vi "Set Parameters.vi"(8 "error in (no error)":errorcluster, 11 "Cluster in":T1={"Queue Array"=[], "Queue Element"={"state"="", "data"=variant}, "System Event"=refnum, "System Event RefNum"=refnum, "Queue List"=[], "LPCA COM"="", "Rotating"=FALSE, "PrecorAI"="", "T_0 Index"=0, "Bar Graph X"=[], "Channels"=[], "Active Indicies"=[], "Active Channels"=[], "Sample Frequency"=0.0, "Ibrake Sweep"=[], "RPM Sweep"=[], "Load Sweep"=[], "Step Height Sweep"=[], "Range Sweep"=[], "A Counter"=0, "B Counter"=0, "C Counter"=0, "#A"=0, "#B"=0, "#C"=0, "Current RPM"=0.0, "Current Ibrake"=0, "Current Range"=0, "Current Step Height"=0, "Load Bank"=enum."OFF", "Cfg Cntrls"=[], "T_Monitor Indices"=[], "Thermal Limit"=0, "Thermal Resume"=0, "Timer Reset"=FALSE, "Stop Time"=0.0, "Autotest"=FALSE, "Pulsed RPM Capture"=FALSE, "Get Sample"=FALSE, "Last State"="", "Reset Timeout"=FALSE, "Ctrl Refs"={"Test Details"=refnum, "Save Config"=refnum, "Load Config"=refnum, "Path"=refnum, "Snapshot"=refnum, "SS#"=refnum, "Ibrake"=refnum, "RPM Target"=refnum, "Spin"=refnum, "Load Bank"=refnum, "Start Test"=refnum, "Pause Test"=refnum, "Load Sweep"=refnum, "RPM Sweep"=refnum, "Ibrake Sweep"=refnum, "Filters"=refnum, "Sample Frequency"=refnum, "Data Setup"=refnum, "Pause"=refnum, "Stop Time"=refnum, "S Period"=refnum, "Range"=refnum, "Step Height"=refnum, "Step Height Sweep"=refnum, "Range Sweep"=refnum, "Available Tests"=refnum, "RPM Graph"=refnum, "RPM Knob"=refnum, "FanMode"=refnum, "Fan Mode LED Array"=refnum, "Thermal Equilibrium"=refnum, "Data Display"=refnum, "LPCA Error"=refnum, "LPCA Ramp"=refnum, "LPCA Range"=refnum, "LPCA Resistance"=refnum, "Analyze Read"=refnum, "Console Select"=refnum, "Sub Panel"=refnum}, "Pulse Waveform"={"t0"=timestamp(0 s since 1904-01-01), "dt"=1.0, "Y"=[]}, "Snapshot"={"Test Details"="test", "Version"="test", "Date"=timestamp(3493915594.3018084 s since 1904-01-01), "Selected Test"="man", "Snapshot Number"=0, "Time"=timestamp(3493915602.7292905 s since 1904-01-01), "Ibrake Setpoint"="1", "RPM Setpoint"="20", "Range Setpoint"="", "Step Height Setpoint"="", "Load Bank Setpoint"="15", "Measurement Headers"="a,b,c,1,2,3", "Measurements"="1,2,3,4,5,6,7,8", "A"=0, "B"=0, "C"=0, "Raw Data"=[], "Available Tests"=enum."Manual", "Ibrake List"="", "RPM List"="", "Load Bank List"="", "Range List"="", "Step Height List"="", "FanMode Setpoint"=enum."Auto"}, "Sample Period"=0.0, "OverTemp"=FALSE, "Available Tests"=enum."Manual", "FanMode"=enum."Auto", "Fan Mode LED Array"=[FALSE, TRUE, FALSE], "Thermal\nEquilibrium "=FALSE, "Equilibrium Stop"=FALSE, "AvgDegChg"=[]} {"Snapshot"."Time" format="%<%H:%M:%S>T"; "Snapshot"."Date" format="%<%m/%d/%Y>T"}) -> (0 "error out":errorcluster, 3 "Cluster out":T1={"Queue Array"=[], "Queue Element"={"state"="", "data"=variant}, "System Event"=refnum, "System Event RefNum"=refnum, "Queue List"=[], "LPCA COM"="", "Rotating"=FALSE, "PrecorAI"="", "T_0 Index"=0, "Bar Graph X"=[], "Channels"=[], "Active Indicies"=[], "Active Channels"=[], "Sample Frequency"=0.0, "Ibrake Sweep"=[], "RPM Sweep"=[], "Load Sweep"=[], "Step Height Sweep"=[], "Range Sweep"=[], "A Counter"=0, "B Counter"=0, "C Counter"=0, "#A"=0, "#B"=0, "#C"=0, "Current RPM"=0.0, "Current Ibrake"=0, "Current Range"=0, "Current Step Height"=0, "Load Bank"=enum."OFF", "Cfg Cntrls"=[], "T_Monitor Indices"=[], "Thermal Limit"=0, "Thermal Resume"=0, "Timer Reset"=FALSE, "Stop Time"=0.0, "Autotest"=FALSE, "Pulsed RPM Capture"=FALSE, "Get Sample"=FALSE, "Last State"="", "Reset Timeout"=FALSE, "Ctrl Refs"={"Test Details"=refnum, "Save Config"=refnum, "Load Config"=refnum, "Path"=refnum, "Snapshot"=refnum, "SS#"=refnum, "Ibrake"=refnum, "RPM Target"=refnum, "Spin"=refnum, "Load Bank"=refnum, "Start Test"=refnum, "Pause Test"=refnum, "Load Sweep"=refnum, "RPM Sweep"=refnum, "Ibrake Sweep"=refnum, "Filters"=refnum, "Sample Frequency"=refnum, "Data Setup"=refnum, "Pause"=refnum, "Stop Time"=refnum, "S Period"=refnum, "Range"=refnum, "Step Height"=refnum, "Step Height Sweep"=refnum, "Range Sweep"=refnum, "Available Tests"=refnum, "RPM Graph"=refnum, "RPM Knob"=refnum, "FanMode"=refnum, "Fan Mode LED Array"=refnum, "Thermal Equilibrium"=refnum, "Data Display"=refnum, "LPCA Error"=refnum, "LPCA Ramp"=refnum, "LPCA Range"=refnum, "LPCA Resistance"=refnum, "Analyze Read"=refnum, "Console Select"=refnum, "Sub Panel"=refnum}, "Pulse Waveform"={"t0"=timestamp(0 s since 1904-01-01), "dt"=1.0, "Y"=[]}, "Snapshot"={"Test Details"="test", "Version"="test", "Date"=timestamp(3493915594.3018084 s since 1904-01-01), "Selected Test"="man", "Snapshot Number"=0, "Time"=timestamp(3493915602.7292905 s since 1904-01-01), "Ibrake Setpoint"="1", "RPM Setpoint"="20", "Range Setpoint"="", "Step Height Setpoint"="", "Load Bank Setpoint"="15", "Measurement Headers"="a,b,c,1,2,3", "Measurements"="1,2,3,4,5,6,7,8", "A"=0, "B"=0, "C"=0, "Raw Data"=[], "Available Tests"=enum."Manual", "Ibrake List"="", "RPM List"="", "Load Bank List"="", "Range List"="", "Step Height List"="", "FanMode Setpoint"=enum."Auto"}, "Sample Period"=0.0, "OverTemp"=FALSE, "Available Tests"=enum."Manual", "FanMode"=enum."Auto", "Fan Mode LED Array"=[FALSE, TRUE, FALSE], "Thermal\nEquilibrium "=FALSE, "Equilibrium Stop"=FALSE, "AvgDegChg"=[]} {"Snapshot"."Time" format="%<%H:%M:%S>T"; "Snapshot"."Date" format="%<%m/%d/%Y>T"})   [LabVIEW 2017]
uses:
  Controls/Test TypeDef.ctl
  Code Library/Queue References Array.ctl
  Code Library/Queue Element.ctl
  Controls/Load Bank.ctl
  Controls/Available Tests.ctl
  Console Sim/Controls/Console Select.ctl
  Controls/Snapshot Typedef.ctl
  Controls/FanMode.ctl
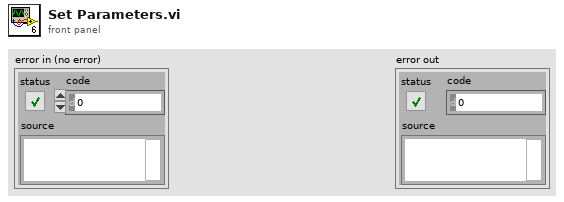
[diagram p1: front panel]
types:
  T1 = typedef "Test TypeDef.ctl" = cluster{"Queue Array":T2, "Queue Element":T3, "System Event":refnum<user-event>, "System Event RefNum":refnum<event-registration>, "Queue List":string[], "LPCA COM":refnum<visa-resource-name>, "Rotating":bool, "PrecorAI":refnum<k21>, "T_0 Index":i32, "Bar Graph X":i32[], "Channels":string[], "Active Indicies":i32[], "Active Channels":string[][], "Sample Frequency":dbl, "Ibrake Sweep":string[], "RPM Sweep":string[], "Load Sweep":string[], "Step Height Sweep":string[], "Range Sweep":string[], "A Counter":i32, "B Counter":i32, "C Counter":i32, "#A":i32, "#B":i32, "#C":i32, "Current RPM":dbl, "Current Ibrake":u32, "Current Range":u32, "Current Step Height":u32, "Load Bank":T4, "Cfg Cntrls":refnum<vi>[], "T_Monitor Indices":i32[], "Thermal Limit":i32, "Thermal Resume":i32, "Timer Reset":bool, "Stop Time":dbl, "Autotest":bool, "Pulsed RPM Capture":bool, "Get Sample":bool, "Last State":string, "Reset Timeout":bool, "Ctrl Refs":cluster{"Test Details":refnum<vi>, "Save Config":refnum<vi>, "Load Config":refnum<vi>, "Path":refnum<vi>, "Snapshot":refnum<vi>, "SS#":refnum<vi>, "Ibrake":refnum<vi>, "RPM Target":refnum<vi>, "Spin":refnum<vi>, "Load Bank":refnum<vi>, "Start Test":refnum<vi>, "Pause Test":refnum<vi>, "Load Sweep":refnum<vi>, "RPM Sweep":refnum<vi>, "Ibrake Sweep":refnum<vi>, "Filters":refnum<vi>, "Sample Frequency":refnum<vi>, "Data Setup":refnum<vi>, "Pause":refnum<vi>, "Stop Time":refnum<vi>, "S Period":refnum<vi>, "Range":refnum<vi>, "Step Height":refnum<vi>, "Step Height Sweep":refnum<vi>, "Range Sweep":refnum<vi>, "Available Tests":refnum<vi>, "RPM Graph":refnum<vi>, "RPM Knob":refnum<vi>, "FanMode":refnum<vi>, "Fan Mode LED Array":refnum<vi>, "Thermal Equilibrium":refnum<vi>, "Data Display":refnum<vi>, "LPCA Error":refnum<vi>, "LPCA Ramp":refnum<vi>, "LPCA Range":refnum<vi>, "LPCA Resistance":refnum<vi>, "Analyze Read":refnum<vi>, "Console Select":refnum<vi>, "Sub Panel":refnum<vi>}, "Pulse Waveform":waveform(dbl), "Snapshot":T5, "Sample Period":dbl, "OverTemp":bool, "Available Tests":T6, "FanMode":T7, "Fan Mode LED Array":bool[], "Thermal\nEquilibrium ":bool, "Equilibrium Stop":bool, "AvgDegChg":dbl[]}
  T2 = typedef "Queue References Array.ctl" = refnum<queue>[]
  T3 = typedef "Queue Element.ctl" = cluster{"state":string, "data":variant}
  T4 = typedef "Load Bank.ctl" = enum16{"OFF", "50", "25", "16.7", "12.5", "10.0", "8.3", "7.1", "6.3", "5.6", "5.0", "4.5", "4.2", "3.8", "3.6", "3.3", "3.1"}
  T5 = typedef "Snapshot Typedef.ctl" = cluster{"Test Details":string, "Version":string, "Date":timestamp, "Selected Test":string, "Snapshot Number":u16, "Time":timestamp, "Ibrake Setpoint":string, "RPM Setpoint":string, "Range Setpoint":string, "Step Height Setpoint":string, "Load Bank Setpoint":string, "Measurement Headers":string, "Measurements":string, "A":i32, "B":i32, "C":i32, "Raw Data":string[][], "Available Tests":T6, "Ibrake List":string, "RPM List":string, "Load Bank List":string, "Range List":string, "Step Height List":string, "FanMode Setpoint":T7}
  T6 = typedef "Available Tests.ctl" = enum16{"Manual", "EFX Brake Torque", "Generator Torque", "EFX Brake Thermal", "Generator Thermal", "Pulsed RPM", "AMT Brake Torque", "Bike Brake Torque", "AMT Brake Thermal", "Bike Brake Thermal"}
  T7 = typedef "FanMode.ctl" = enum16{"On", "Off", "Auto"}
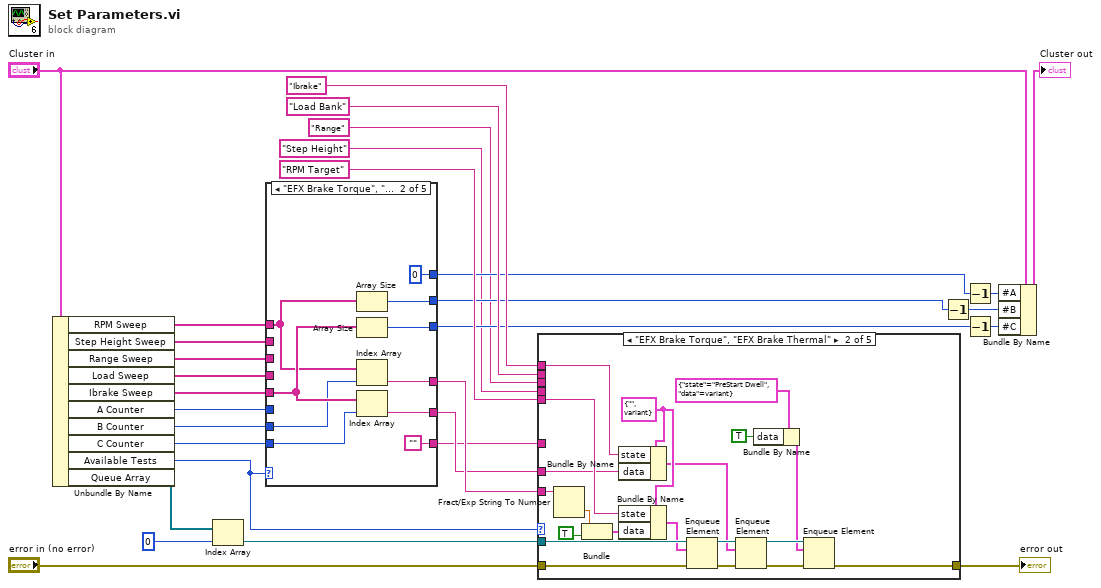
[diagram p0: block diagram]
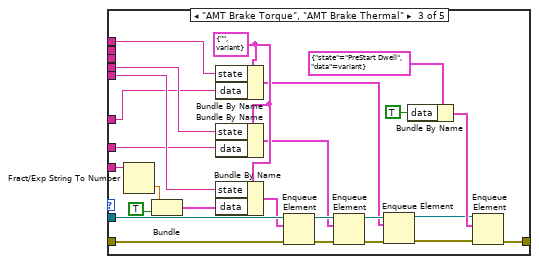
[diagram p3: hidden frame]
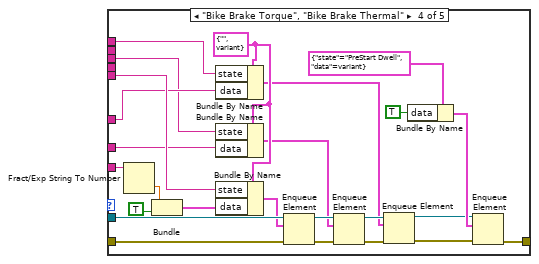
[diagram p4: hidden frame]
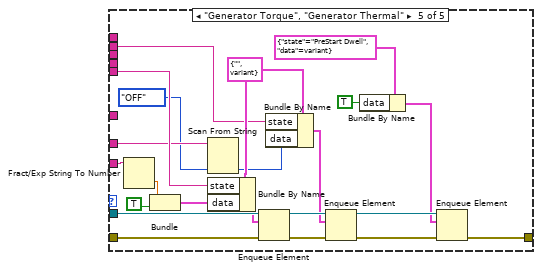
[diagram p5: hidden frame]
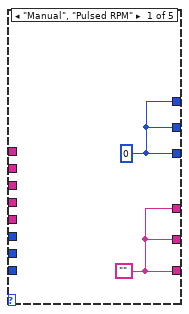
[diagram p6: hidden frame]
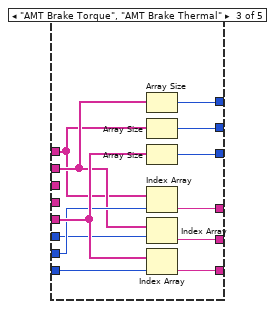
[diagram p7: hidden frame]
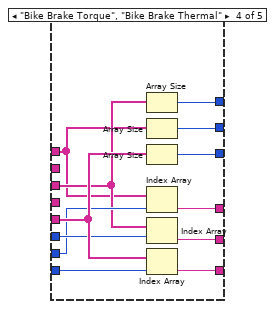
[diagram p8: hidden frame]
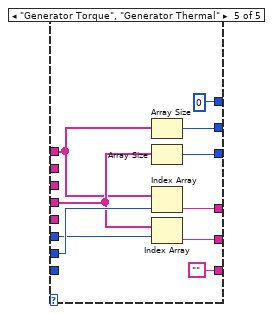
[diagram p9: hidden frame]
diagram:
  n1 = Unbundle By Name("Cluster in") -> ("RPM Sweep"=w19:string[], "Step Height Sweep"=w20:string[], "Range Sweep"=w21:string[], "Load Sweep"=w11:string[], "Ibrake Sweep"=w10:string[], "A Counter"=w17:i32, "B Counter"=w18:i32, "C Counter"=w9:i32, "Available Tests"=w26:T6, "Queue Array"=w24:T2)
  n2 = Index Array(array=w24, index=0) -> (element=w25:refnum<queue>)
  n3 = case shown="\"EFX Brake Torque\", \"EFX Brake Thermal\"" w26 {
    tunnel: w19 -> [_ w39 w46 w55 w71]
    tunnel: w20 -> [_ _ w47 _ _]
    tunnel: w21 -> [_ _ _ w56 _]
    tunnel: w17 -> [_ _ w48 w58 w73]
    tunnel: w18 -> [_ w34 w49 w57 w74]
    tunnel: [w32 w41 w54 w66 w75] -> w2
    tunnel: [w32 w42 w53 w65 w76] -> w3
    tunnel: [w31 w37 w45 w64 w69] -> w7
    tunnel: [w31 0 w43 w63 0] -> w6
    tunnel: w11 -> [_ _ _ _ w72]
    tunnel: w10 -> [_ w40 w51 w61 _]
    tunnel: w9 -> [_ w33 w52 w62 _]
    tunnel: [w31 w36 w44 w60 w68] -> w8
    tunnel: [w32 "" w50 w59 ""] -> w1
    frame "Manual", "Pulsed RPM" {
      w31 = 0
      w32 = ""
    }
    frame "EFX Brake Torque", "EFX Brake Thermal" {
      n4 = Array Size(array=w39) -> (size(s)=w37:i32)
      n5 = Array Size(array=w40) -> (size(s)=w36:i32)
      n6 = Index Array(array=w39, index=w34) -> (element=w42:string)
      n7 = Index Array(array=w40, index=w33) -> (element=w41:string)
    }
    frame "AMT Brake Torque", "AMT Brake Thermal" {
      n8 = Array Size(array=w47) -> (size(s)=w43:i32)
      n9 = Array Size(array=w46) -> (size(s)=w45:i32)
      n10 = Array Size(array=w51) -> (size(s)=w44:i32)
      n11 = Index Array(array=w46, index=w49) -> (element=w53:string)
      n12 = Index Array(array=w47, index=w48) -> (element=w54:string)
      n13 = Index Array(array=w51, index=w52) -> (element=w50:string)
    }
    frame "Bike Brake Torque", "Bike Brake Thermal" {
      n14 = Array Size(array=w56) -> (size(s)=w63:i32)
      n15 = Array Size(array=w55) -> (size(s)=w64:i32)
      n16 = Array Size(array=w61) -> (size(s)=w60:i32)
      n17 = Index Array(array=w55, index=w57) -> (element=w65:string)
      n18 = Index Array(array=w56, index=w58) -> (element=w66:string)
      n19 = Index Array(array=w61, index=w62) -> (element=w59:string)
    }
    frame "Generator Torque", "Generator Thermal" {
      n20 = Array Size(array=w71) -> (size(s)=w69:i32)
      n21 = Array Size(array=w72) -> (size(s)=w68:i32)
      n22 = Index Array(array=w71, index=w74) -> (element=w76:string)
      n23 = Index Array(array=w72, index=w73) -> (element=w75:string)
    }
  }
  n24 = case shown="\"EFX Brake Torque\", \"EFX Brake Thermal\"" w26 {
    tunnel: "error in (no error)" -> [w77 w96 w121 w146 w168]
    tunnel: [w77 w81 w111 w136 w153] -> w13
    tunnel: w25 -> [_ w95 w120 w145 w167]
    tunnel: "RPM Target" -> [_ w92 w117 w142 w164]
    tunnel: w3 -> [_ w91 w116 w141 w163]
    tunnel: "Load Bank" -> [_ _ _ _ w160]
    tunnel: w2 -> [_ w88 w104 w129 w156]
    tunnel: "Ibrake" -> [_ w84 w112 w137 _]
    tunnel: "Step Height" -> [_ _ w102 _ _]
    tunnel: "Range" -> [_ _ _ w123 _]
    tunnel: w1 -> [_ _ w101 w127 _]
    frame "Manual", "Pulsed RPM" {
    }
    frame "EFX Brake Torque", "EFX Brake Thermal" {
      w90 = T3 {"state"="", "data"=variant} ("element")
      n25 = Fract/Exp String To Number(string=w91) -> (number=w85:dbl)  [unwired: 3 in, 1 out]
      n26 = Bundle(w85, TRUE) -> (w87:cluster{dbl, bool})  [unwired: 1 in]
      n27 = Bundle By Name(cluster=w90, "state"=w84, "data"=w88) -> (w89:T3)
      n28 = Bundle By Name(cluster=w90, "state"=w92, "data"=w87) -> (w93:T3)
      n29 = Enqueue Element(queue=w95, element=w93, error in (no error)=w96) -> (queue out=w94:refnum<queue>, error out=w97:errorcluster)  [unwired: 1 in, 1 out]
      n30 = Enqueue Element(queue=w94, element=w89, error in (no error)=w97) -> (queue out=w83:refnum<queue>, error out=w82:errorcluster)  [unwired: 1 in, 1 out]
      n31 = Bundle By Name(cluster=T3 {"state"="PreStart Dwell", "data"=variant} ("element"), "data"=TRUE) -> (w79:T3)
      n32 = Enqueue Element(queue=w83, element=w79, error in (no error)=w82) -> (error out=w81:errorcluster)  [unwired: 1 in, 2 out]
    }
    frame "AMT Brake Torque", "AMT Brake Thermal" {
      w105 = T3 {"state"="", "data"=variant} ("element")
      n33 = Fract/Exp String To Number(string=w116) -> (number=w113:dbl)  [unwired: 3 in, 1 out]
      n34 = Bundle(w113, TRUE) -> (w115:cluster{dbl, bool})  [unwired: 1 in]
      n35 = Bundle By Name(cluster=w105, "state"=w112, "data"=w101) -> (w100:T3)
      n36 = Bundle By Name(cluster=w105, "state"=w102, "data"=w104) -> (w103:T3)
      n37 = Bundle By Name(cluster=w105, "state"=w117, "data"=w115) -> (w118:T3)
      n38 = Enqueue Element(queue=w120, element=w118, error in (no error)=w121) -> (queue out=w119:refnum<queue>, error out=w122:errorcluster)  [unwired: 1 in, 1 out]
      n39 = Enqueue Element(queue=w119, element=w103, error in (no error)=w122) -> (queue out=w107:refnum<queue>, error out=w99:errorcluster)  [unwired: 1 in, 1 out]
      n40 = Enqueue Element(queue=w107, element=w100, error in (no error)=w99) -> (queue out=w106:refnum<queue>, error out=w98:errorcluster)  [unwired: 1 in, 1 out]
      n41 = Bundle By Name(cluster=T3 {"state"="PreStart Dwell", "data"=variant} ("element"), "data"=TRUE) -> (w109:T3)
      n42 = Enqueue Element(queue=w106, element=w109, error in (no error)=w98) -> (error out=w111:errorcluster)  [unwired: 1 in, 2 out]
    }
    frame "Bike Brake Torque", "Bike Brake Thermal" {
      w130 = T3 {"state"="", "data"=variant} ("element")
      n43 = Fract/Exp String To Number(string=w141) -> (number=w138:dbl)  [unwired: 3 in, 1 out]
      n44 = Bundle(w138, TRUE) -> (w140:cluster{dbl, bool})  [unwired: 1 in]
      n45 = Bundle By Name(cluster=w130, "state"=w137, "data"=w127) -> (w126:T3)
      n46 = Bundle By Name(cluster=w130, "state"=w123, "data"=w129) -> (w128:T3)
      n47 = Bundle By Name(cluster=w130, "state"=w142, "data"=w140) -> (w143:T3)
      n48 = Enqueue Element(queue=w145, element=w143, error in (no error)=w146) -> (queue out=w144:refnum<queue>, error out=w147:errorcluster)  [unwired: 1 in, 1 out]
      n49 = Enqueue Element(queue=w144, element=w128, error in (no error)=w147) -> (queue out=w132:refnum<queue>, error out=w125:errorcluster)  [unwired: 1 in, 1 out]
      n50 = Enqueue Element(queue=w132, element=w126, error in (no error)=w125) -> (queue out=w131:refnum<queue>, error out=w124:errorcluster)  [unwired: 1 in, 1 out]
      n51 = Bundle By Name(cluster=T3 {"state"="PreStart Dwell", "data"=variant} ("element"), "data"=TRUE) -> (w134:T3)
      n52 = Enqueue Element(queue=w131, element=w134, error in (no error)=w124) -> (error out=w136:errorcluster)  [unwired: 1 in, 2 out]
    }
    frame "Generator Torque", "Generator Thermal" {
      w162 = T3 {"state"="", "data"=variant} ("element")
      n53 = Fract/Exp String To Number(string=w163) -> (number=w157:dbl)  [unwired: 3 in, 1 out]
      n54 = Bundle(w157, TRUE) -> (w159:cluster{dbl, bool})  [unwired: 1 in]
      n55 = Scan From String(input string=w156, default 1=Load_Bank."OFF" ("Load Bank")) -> (output 1=w155:T4)  [unwired: 3 in, 3 out]
      n56 = Bundle By Name(cluster=w162, "state"=w164, "data"=w159) -> (w165:T3)
      n57 = Enqueue Element(queue=w167, element=w165, error in (no error)=w168) -> (queue out=w166:refnum<queue>, error out=w169:errorcluster)  [unwired: 1 in, 1 out]
      n58 = Bundle By Name(cluster=w162, "state"=w160, "data"=w155) -> (w161:T3)
      n59 = Enqueue Element(queue=w166, element=w161, error in (no error)=w169) -> (queue out=w152:refnum<queue>, error out=w154:errorcluster)  [unwired: 1 in, 1 out]
      n60 = Bundle By Name(cluster=T3 {"state"="PreStart Dwell", "data"=variant} ("element"), "data"=TRUE) -> (w148:T3)
      n61 = Enqueue Element(queue=w152, element=w148, error in (no error)=w154) -> (error out=w153:errorcluster)  [unwired: 1 in, 2 out]
    }
  }
  "error out" <- w13
  n62 = Decrement(x=w7) -> (x-1=w29:i32)
  n63 = Decrement(x=w6) -> (x-1=w28:i32)
  n64 = Decrement(x=w8) -> (x-1=w12:i32)
  n65 = Bundle By Name(cluster="Cluster in", "#A"=w28, "#B"=w29, "#C"=w12) -> (→"Cluster out":T1)
